vi "Mute All.vi"(8 "Error In":errorcluster, 10 "Mute All":bool, 11 "KIT-QVA in":refnum<class "KIT-QVA.lvclass">) -> (0 "Error Out":errorcluster, 3 "KIT-QVA out":refnum<class "KIT-QVA.lvclass">)   [LabVIEW 2016, in "KIT-QVA.lvlib" / "KIT-QVA.lvclass"]
doc: "Activate or deactivate time unlimited muting of all, marked and unmarked, detectors."
uses:
  KIT-QVA.lvclass
  KIT-QVA.lvclass/KIT-QVA.ctl
  instr.lib/KIT-QV/KIT QV.lvlib
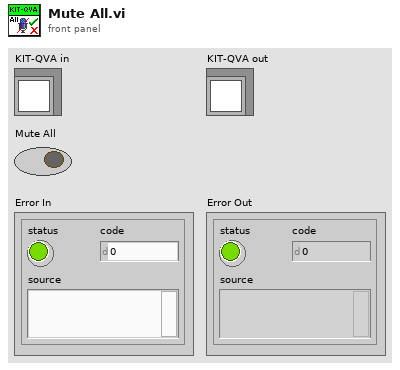
[diagram p1: front panel]
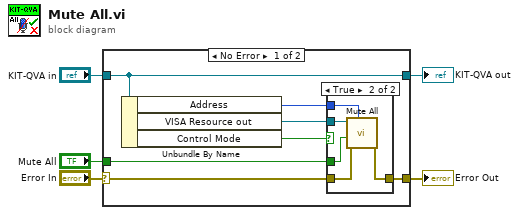
[diagram p0: block diagram]
diagram:
  n1 = case shown="No Error" "Error In" {
    selector: "Error In" -> [w9 w20]
    tunnel: [w8 w20] -> w4
    tunnel: [w12 w19] -> w2
    tunnel: "KIT-QVA in" -> [w12 w19]
    tunnel: "Mute All" -> [w7 _]
    frame No Error {
      n2 = Unbundle By Name(w12) -> ("Address"=w10:u16, "VISA Resource out"=w11:refnum<visa-resource-name>, "Control Mode"=w6:bool)
      n3 = case shown="True" w6 {
        tunnel: w11 -> [_ w18]
        tunnel: w10 -> [_ w17]
        tunnel: w9 -> [w13 w16]
        tunnel: w7 -> [_ w14]
        tunnel: [w13 w15] -> w8
        frame False {
        }
        frame True {
          n4 = call "Mute All.vi"("Address"=w17, "Error In"=w16, "Mute All (F)"=w14, "VISA Resource in"=w18) -> ("Error Out"=w15:errorcluster)  [unwired: 6 in, 1 out]
        }
      }
    }
    frame Error {
    }
  }
  "Error Out" <- w4
  "KIT-QVA out" <- w2
